vi "Save for Previous Version.vi"(8 "error in (no error)":errorcluster, 10 "LabVIEW Version":string, 11 "LabVIEW File in":refnum<class "LabVIEW File.lvclass">) -> (0 "error out":errorcluster, 1 "Errors":string, 2 "Warnings":string, 3 "LabVIEW File out":refnum<class "LabVIEW File.lvclass">)   [LabVIEW 2020, in "Save for Previous Version.lvlib" / "LabVIEW File.lvclass"]
uses:
  LabVIEW File.lvclass
  LabVIEW File.lvclass/LabVIEW File.ctl
  Read Version String.vi
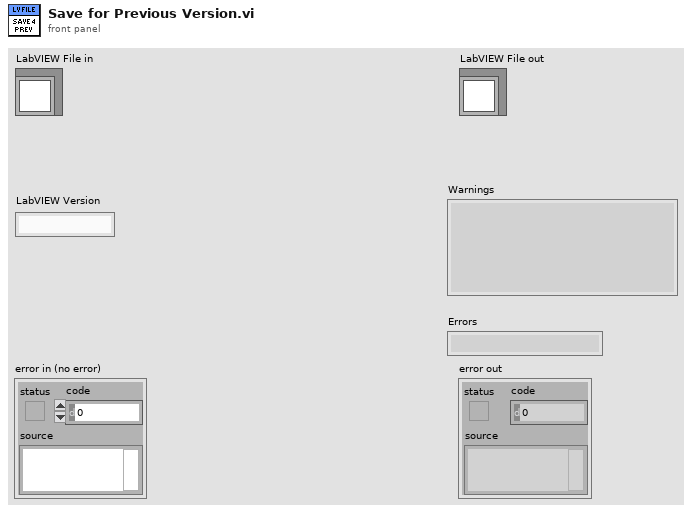
[diagram p1: front panel]
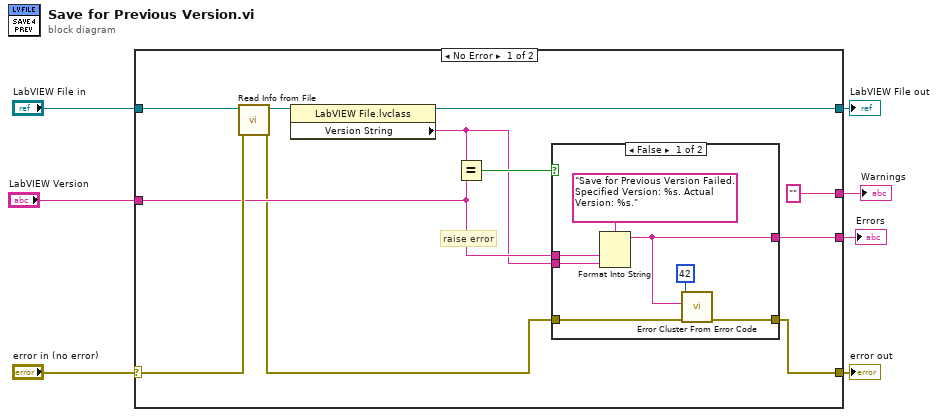
[diagram p0: block diagram]
diagram:
  n1 = case shown="No Error" "error in (no error)" {
    selector: "error in (no error)" -> [w17 w28]
    tunnel: [w15 w28] -> w6
    tunnel: [w16 w27] -> w4
    tunnel: "LabVIEW File in" -> [w18 w27]
    tunnel: "LabVIEW Version" -> [w14 _]
    tunnel: [w13 _] -> w2
    tunnel: ["" ("Warnings") _] -> w1
    frame No Error {
      # "raise error"
      n2 = call-dynamic "Read Info from File.vi"("error in (no error)"=w17, "LabVIEW File in"=w18) -> ("error out"=w9:errorcluster, "LabVIEW File out"=w11:refnum<class "LabVIEW File.lvclass">)  [unwired: 8 in]
      n3 = property class="LabVIEW File.lvclass"(reference=w11) -> (reference out=w16:refnum<class "LabVIEW File.lvclass">, "Version String"=w8:string)  [unwired: 1 in, 1 out]
      n4 = Equal?(x=w8, y=w14) -> (x = y?=w10:bool)
      n5 = case shown="False" w10 {
        tunnel: [w25 w26] -> w15
        tunnel: w9 -> [w24 w26]
        tunnel: w14 -> [w22 _]
        tunnel: w8 -> [w21 _]
        tunnel: [w19 _] -> w13
        frame False {
          n6 = Format Into String(format string="Save for Previous Version Failed. Specified Version: %s. Actual Version: %s.", w22, w21) -> (resulting string=w19:string)  [unwired: 2 in, 1 out]
          n7 = call <vilib>:"Error Cluster From Error Code.vi"("error in (no error)"=w24, "error message (\"\")"=w19, "error code (0)"=42) -> ("error out"=w25:errorcluster)  [unwired: 6 in]
        }
        frame True {
        }
      }
    }
    frame Error {
    }
  }
  "error out" <- w6
  "LabVIEW File out" <- w4
  "Warnings" <- w1
  "Errors" <- w2
